vi "MakeInterLock.vi"(1 "Interlock Name":string, 2 "Interlock Ready":bool=TRUE) -> (0 "Interlock Unit":T1={"Interlock State"=TRUE, "Interlock Name"=""})   [LabVIEW 2016]
uses:
  InterlockElement.ctl
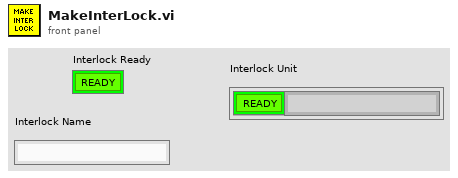
[diagram p1: front panel]
types:
  T1 = typedef "InterlockElement.ctl" = cluster{"Interlock State":bool, "Interlock Name":string}
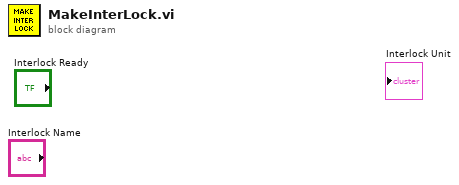
[diagram p0: block diagram]
diagram:
